vi "BRig_dataAnalog_valueAI1_1.vi"() -> (2 "output_valueAI1_1":i32)   [LabVIEW 2014]
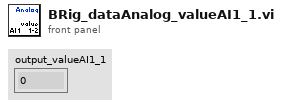
[diagram p1: front panel]
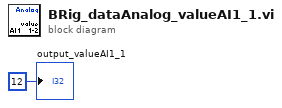
[diagram p0: block diagram]
diagram:
  "output_valueAI1_1" <- 12 ("output_iBlock")
